vi "Read Children Symbol Information.vi"(6 "Get all descendents?":bool, 8 "error in (no error)":errorcluster, 10 "Parent Name":string, 11 "TwinCAT ADS in":refnum<class "TwinCAT ADS.lvclass">) -> (0 "error out":errorcluster, 1 "Symbols Information":T1[](array[typedef]) {"Type ID" items=["ADST_VOID"=0, "ADST_INT16"=2, "ADST_INT32"=3, "ADST_REAL32"=4, "ADST_REAL64"=5, "ADST_INT8"=16, "ADST_UINT8"=17, "ADST_UINT16"=18, "ADST_UINT32"=19, "ADST_INT64"=20, "ADST_UINT64"=21, "ADST_STRING"=30, "ADST_WSTRING"=31, "ADST_REAL80"=32, "ADST_BIT"=33, "ADST_MAXTYPES"=34, "ADST_BIGTYPE"=65]; "Type Category" items=["Unknown, None"=0, "Primitive"=1, "Alias"=2, "Enum"=3, "Array"=4, "Struct"=5, "FunctionBlock"=6, "Program"=7, "Function"=8, "SubRange"=9, "String"=10, "Bitset"=12, "Pointer"=13, "Union"=14, "Reference"=15, "Interface"=16]}, 3 "TwinCAT ADS out":refnum<class "TwinCAT ADS.lvclass">)   [LabVIEW 2018, in "TwinCAT ADS.lvclass"]
uses:
  TwinCAT ADS.lvclass
  Controls/Symbol Information.ctl
  TwinCAT.Ads
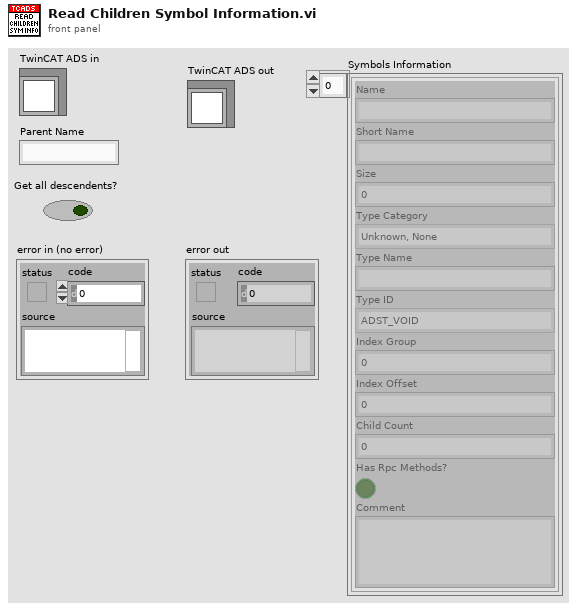
[diagram p1: front panel]
types:
  T1 = typedef "TwinCAT ADS.lvclass/Symbol Information.ctl" = cluster{"Name":string, "Short Name":string, "Size":i32, "Type Category":i32, "Type Name":string, "Type ID":i32, "Index Group":i64, "Index Offset":i64, "Child Count":i32, "Has Rpc Methods?":bool, "Comment":string}
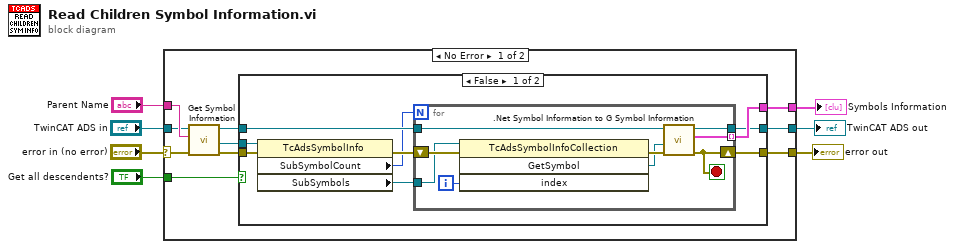
[diagram p0: block diagram]
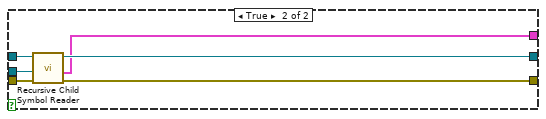
[diagram p2: hidden frame]
diagram:
  n1 = case shown="No Error" "error in (no error)" {
    selector: "error in (no error)" -> [w17 w43]
    tunnel: [w12 w43] -> w2
    tunnel: [w13 w42] -> w1
    tunnel: "TwinCAT ADS in" -> [w8 w42]
    tunnel: "Parent Name" -> [w16 _]
    tunnel: [w14 _] -> w3
    tunnel: "Get all descendents?" -> [w11 _]
    frame No Error {
      n2 = call-dynamic "Get Symbol Information.vi"("error in (no error)"=w17, "Name"=w16, "TwinCAT ADS in"=w8) -> ("error out"=w10:errorcluster, "Symbol Info"=w9:refnum<k24>, "TwinCAT ADS out"=w15:refnum<class "TwinCAT ADS.lvclass">)  [unwired: 6 in]
      n3 = case shown="False" w11 {
        tunnel: w10 -> [w24 w41]
        tunnel: w15 -> [w21 w40]
        tunnel: [w26 w36] -> w14
        tunnel: [w18 w38] -> w13
        tunnel: [w25 w37] -> w12
        tunnel: w9 -> [w22 w39]
        frame False {
          n4 = property class="TcAdsSymbolInfo"(reference=w22, error in=w24) -> (error out=w23:errorcluster, "SubSymbolCount"=w20:i32, "SubSymbols"=w19:refnum<k24>)  [unwired: 1 out]
          n5 = for {
            N: w20 -> [_]
            shift-right: [w27] -> w25
            shift-left: w23 -> [w33]
            tunnel: [w30] -> w26 mode=indexing
            tunnel: w19 -> [w32]
            tunnel: w21 -> [w29]
            tunnel: [w28] -> w18
            i -> [w34]
            stop <- w27 stop-if-true
            n6 = invoke class="TcAdsSymbolInfoCollection" method="GetSymbol"(reference=w32, error in=w33, "index"=w34) -> (error out=w35:errorcluster, "GetSymbol"=w31:refnum<k24>)  [unwired: 1 in, 2 out]
            n7 = call ".Net Symbol Information to G Symbol Information.vi"("TwinCAT ADS in"=w29, ".NET ITcAdsSymbolInfo refnum"=w31, "error in (no error)"=w35) -> ("TwinCAT ADS out"=w28:refnum<class "TwinCAT ADS.lvclass">, "Symbol Information"=w30:T1, "error out"=w27:errorcluster)  [unwired: 5 in]
          }
        }
        frame True {
          n8 = call "Recursive Child Symbol Reader.vi"("error in (no error)"=w41, ".NET TcAdsSymbolInfo"=w39, "TwinCAT ADS in"=w40) -> ("error out"=w37:errorcluster, "Symbols Information"=w36:T1[], "TwinCAT ADS out"=w38:refnum<class "TwinCAT ADS.lvclass">)  [unwired: 6 in]
        }
      }
    }
    frame Error {
    }
  }
  "error out" <- w2
  "TwinCAT ADS out" <- w1
  "Symbols Information" <- w3
